vi "Close.vi"(8 "error in (no error)":errorcluster, 11 "IviFgen in":refnum<class "IviFgen.lvclass">) -> (0 "error out":errorcluster, 3 "IviFgen out":refnum<class "IviFgen.lvclass">)   [LabVIEW 2014, in "FgenPlugins.lvlib" / "IviFgen.lvclass"]
uses:
  IviFgen.lvclass
  FgenPluginBaseClass/FgenPluginsBase.lvclass/FgenPluginsBase.ctl
  FgenPluginBaseClass/Accessors/Read Channels.vi
  FgenPluginBaseClass/Accessors/Write Channels.vi
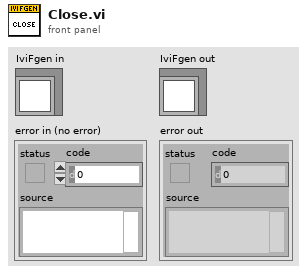
[diagram p1: front panel]
types:
  T1 = typedef "Channel.ctl" = cluster{"Name":string, "Enabled":bool, "Operation":enum16{"Continuous", "Burst"}, "Impedance (50)":dbl, "Handle":string, "Connected":bool, "Mode (Function)":enum16{"Function", "Arbitrary", "Sequence"}}
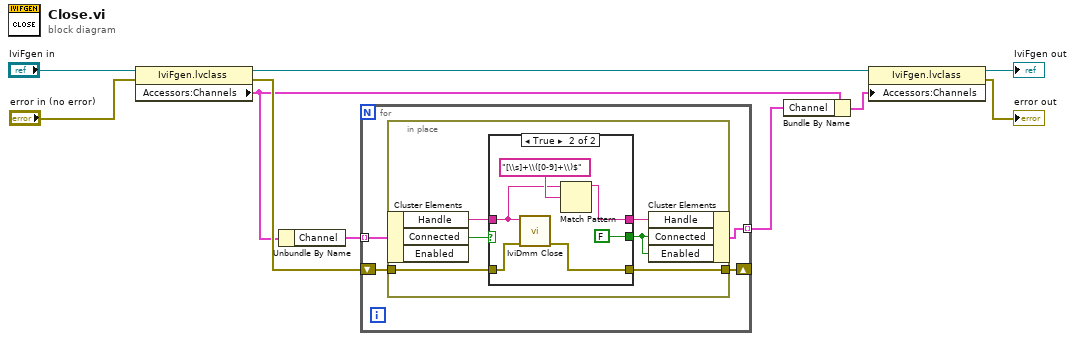
[diagram p0: block diagram]
diagram:
  n1 = property class="IviFgen.lvclass"(reference="IviFgen in", error in="error in (no error)") -> (reference out=w6:refnum<class "IviFgen.lvclass">, error out=w7:errorcluster, "Accessors:Channels"=w3:cluster{"Count":u16, "Channel":T1[]})
  n2 = Unbundle By Name(w3) -> ("Channel"=w8:T1[])
  n3 = for {
    tunnel: w8 -> [w14] mode=indexing
    shift-right: [w12] -> _
    shift-left: w7 -> [w13]
    tunnel: [w11] -> w2 mode=indexing
    n4 = in-place {
      in-place-border: w13 -> [w18]
      in-place-border: [w16] -> w12
      n5 = in-place-cluster #1(w14) -> ("Handle"=w19:string, "Connected"=w20:bool)  [unwired: 1 out]
      n6 = case shown="True" w20 {
        selector: w20 -> [w21 _]
        tunnel: w19 -> [w22 w26]
        tunnel: w18 -> [w23 w29]
        tunnel: [w23 w28] -> w16
        tunnel: [w22 w25] -> w17
        tunnel: [w21 FALSE] -> w15
        frame False {
        }
        frame True {
          n7 = call <vilib>:"IviDmm Close.vi"("error in (no error)"=w29, "instrument handle"=w26) -> ("error out"=w28:errorcluster)  [unwired: 9 in]
          n8 = Match Pattern(string=w26, regular expression="[\\s]+\\([0-9]+\\)$") -> (before substring=w25:string)  [unwired: 1 in, 3 out]
        }
      }
      n9 = in-place-cluster #1("Handle"=w17, "Connected"=w15, "Enabled"=w15) -> (w11:T1)
    }
  }
  n10 = Bundle By Name(cluster=w3, "Channel"=w2) -> (w1:cluster{"Count":u16, "Channel":T1[]})
  n11 = property class="IviFgen.lvclass"(reference=w6, "Accessors:Channels"=w1) -> (reference out=→"IviFgen out":refnum<class "IviFgen.lvclass">, error out=→"error out":errorcluster)  [unwired: 1 in]
